vi "调用命令.vi"(8 "error in (no error)":errorcluster caption="错误输入（无错误）", 11 "控制盒（队列） 输入":refnum<class "控制盒（队列）.lvclass"> caption="DNL_LabVIEW Object in") -> (0 "error out":errorcluster caption="错误输出", 3 "控制盒（队列） 输出":refnum<class "控制盒（队列）.lvclass"> caption="DNL_LabVIEW Object out")   [LabVIEW 2011, in "控制盒（队列）.lvclass"]
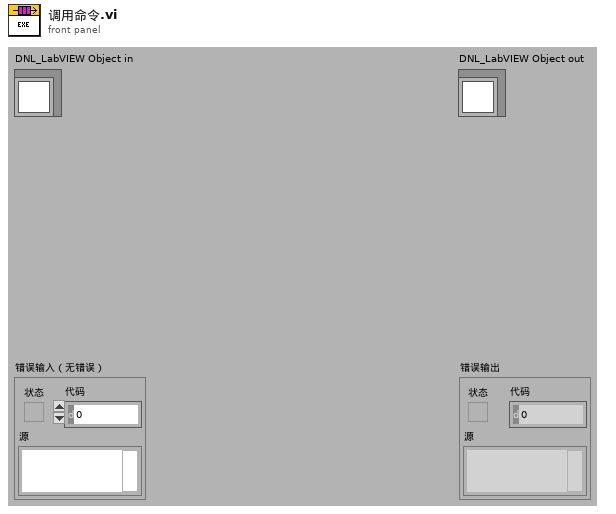
[diagram p1: front panel]
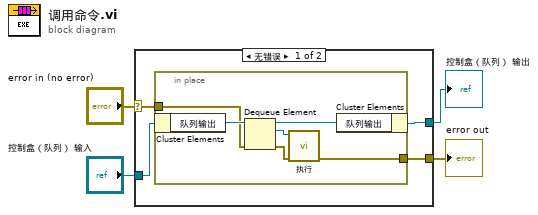
[diagram p0: block diagram]
diagram:
  n1 = case shown="无错误" "error in (no error)" {
    selector: "error in (no error)" -> [w7 w16]
    tunnel: [w6 w16] -> w3
    tunnel: [w5 w15] -> w1
    tunnel: "控制盒（队列） 输入" -> [w8 w15]
    frame No Error {
      n2 = in-place {
        in-place-border: w7 -> [w13]
        in-place-border: [w9] -> w6
        n3 = in-place-cluster #1(w8) -> ("队列输出"=w14:refnum<queue>)
        n4 = Dequeue Element(queue=w14, error in (no error)=w13) -> (queue out=w11:refnum<queue>, element=w12:refnum<class "命令类.lvclass">, error out=w10:errorcluster)  [unwired: 1 in, 1 out]
        n5 = call-dynamic "执行.vi"("error in (no error)"=w10, "命令类 输入"=w12) -> ("error out"=w9:errorcluster)  [unwired: 8 in, 1 out]
        n6 = in-place-cluster #1("队列输出"=w11) -> (w5:refnum<class "控制盒（队列）.lvclass">)
      }
    }
    frame Error {
    }
  }
  "error out" <- w3
  "控制盒（队列） 输出" <- w1
